vi "JSON to Anything.vi"(8 "error in (no error)":errorcluster, 9 "Error on Mismatch (F)":bool, 10 "JSON Object":string, 11 "Type":variant) -> (0 "error out":errorcluster, 1 "Mismatch":bool, 2 "Variant Data String":string, 3 "Variant":variant)   [LabVIEW 2011, in "LV JSON.lvlib"]
doc: "Load values from JSON Object into LabVIEW data type. If key names don't match, defaults will be used.\n\nVariant Data String is used for recusion only."
uses:
  LV JSON.lvlib
  <vilib>/Utility/VariantDataType/Type.ctl
  subVIs/Scan Bracketed String.vi
  subVIs/JSON Type.vi
  <vilib>/Utility/error.llb/Trim Whitespace.vi
  <vilib>/Utility/VariantDataType/VariantType.lvlib
panel:
  out "Type Enum":T1
  # "These indicators are for debug only"
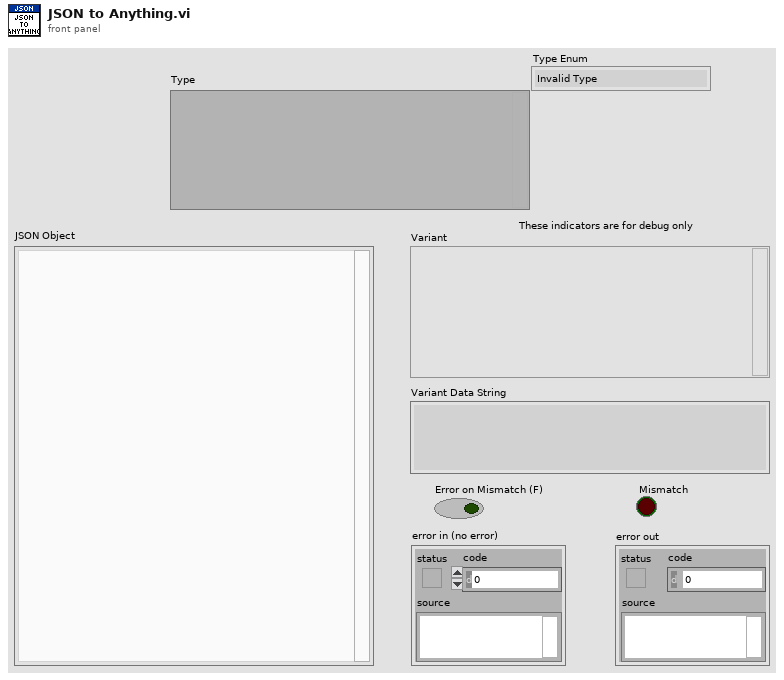
[diagram p1: front panel]
types:
  T1 = typedef "VariantType.lvlib/Type.ctl" = enum8{"Invalid Type", "Void", "I8", "I16", "I32", "I64", "U8", "U16", "U32", "U64", "Single Float", "Double Float", "Extended Float", "Single Complex", "Double Complex", "Extended Complex", "Enum U8", "Enum U16", "Enum U32", "Enum U64", "Single Float With Unit", "Double Float With Unit", "Extended Float With Unit", "Single Complex with Unit", "Double Complex with Unit", "Extended Complex with Unit", "Boolean", "String", "Path", "Picture", "Tag", "Array", "Cluster", "Variant", "LV Variant", "Waveform", "Timestamp", "Digital Waveform", "Digital Data", "ExpressData", "Refnum", "External Data", "VI", "Poly VI", "LabVIEW Class Instance", "Fixed Point"}
  T2 = typedef "LV JSON.lvlib/JSON type.ctl" = enum16{"object", "array", "number", "string", "boolean", "null"}
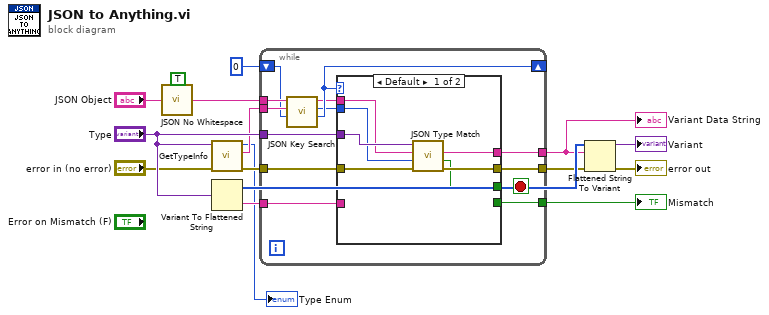
[diagram p0: block diagram]
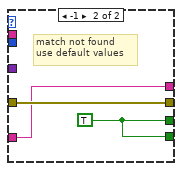
[diagram p2: hidden frame]
diagram:
  n1 = call "JSON No Whitespace.vi"("String"="JSON Object", "Except in Quotes (F)"=TRUE) -> ("Trimmed String"=w1:string)
  n2 = call <vilib>:"GetTypeInfo.vi"("error in (no error)"="error in (no error)", "Variant"="Type") -> ("error out"=w13:errorcluster, "Name"=w11:string, "Type Enum"=→"Type Enum":T1)  [unwired: 5 in, 2 out]
  n3 = Variant To Flattened String(Variant="Type") -> (data string=w5:string, 1:w14:i16[])
  n4 = while {
    tunnel: w13 -> [w29]
    tunnel: "Type" -> [w28]
    tunnel: w1 -> [w27]
    tunnel: w11 -> [w26]
    shift-right: [w23] -> _
    shift-left: 0 ("offset of match") -> [w25]
    tunnel: [w20] -> w7
    tunnel: [w19] -> w8
    tunnel: [w18] -> w6
    tunnel: w5 -> [w17]
    stop <- w24 stop-if-true
    n5 = call "JSON Key Search.vi"("offset (0)"=w25, "Key"=w26, "JSON"=w27) -> ("offset of match"=w23:i32, "JSON Type"=w21:T2, "Value"=w22:string)  [unwired: 6 in]
    n6 = case shown="Default" w23 {
      tunnel: w29 -> [w36 w39]
      tunnel: w28 -> [w34 _]
      tunnel: [w30 w38] -> w24
      tunnel: w22 -> [w33 _]
      tunnel: w21 -> [w32 _]
      tunnel: [w35 w39] -> w20
      tunnel: [w31 w37] -> w19
      tunnel: [_ w38] -> w18
      tunnel: w17 -> [_ w37]
      frame Default {
        n7 = call "JSON Type Match.vi"("error in (no error)"=w36, "JSON Type"=w32, "JSON Value"=w33, "Type"=w34) -> ("error out"=w35:errorcluster, "Types Match"=w30:bool, "Variant Data String"=w31:string)  [unwired: 5 in]
      }
      frame -1 {
        w38 = TRUE
        # "match not found\nuse default values"
      }
    }
  }
  "Mismatch" <- w6
  "Variant Data String" <- w8
  n8 = Flattened String To Variant(4:w7, 6:w8, 7:w14) -> (0:→"error out":errorcluster, 3:→"Variant":variant)
